vi "Verify Directory Exists and Create Tree if Necessary.vi"(0 "path":path=path "C:/Reports", 11 "error in":errorcluster) -> (4 "dup path":path=path "C:/Reports", 15 "error out":errorcluster)   [LabVIEW 2023]
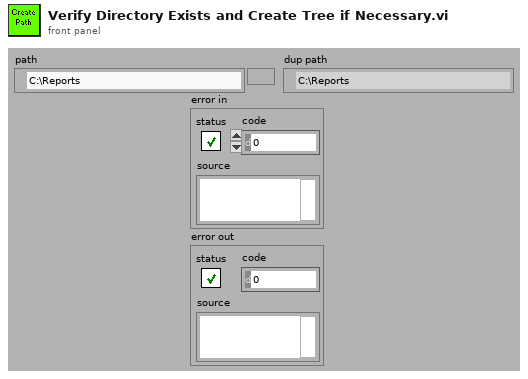
[diagram p1: front panel]
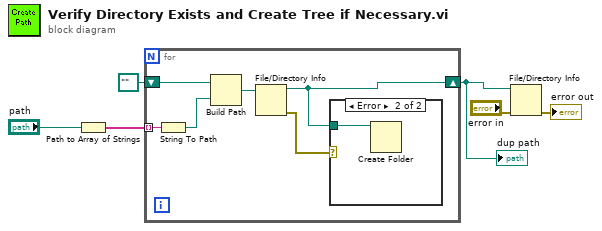
[diagram p0: block diagram]
diagram:
  n1 = Path to Array of Strings(0:"path") -> (2:w5:string[])  [unwired: 1 out]
  n2 = for {
    tunnel: w5 -> [w12] mode=indexing
    shift-right: [w7] -> w1
    shift-left: path "" -> [w10]
    n3 = String To Path(string=w12) -> (path=w9:path)
    n4 = Build Path(base path=w10, name or relative path=w9) -> (appended path=w11:path)
    n5 = File/Directory Info(path=w11) -> (path out=w7:path, error out=w8:errorcluster)  [unwired: 1 in, 5 out]
    n6 = case shown="Error" w8 {
      tunnel: w7 -> [_ w13]
      frame No Error {
      }
      frame Error {
        n7 = Create Folder(path (use dialog)=w13) -> ()  [unwired: 2 in, 3 out]
      }
    }
  }
  "dup path" <- w1
  n8 = File/Directory Info(path=w1, error in="error in") -> (error out=→"error out":errorcluster)  [unwired: 6 out]
